vi "AssignAndCount60_Simple.vi"(7 "Area bits in":bool[](array[boolean])=[FALSE, FALSE, FALSE, FALSE, FALSE, FALSE, FALSE, FALSE, FALSE, FALSE, FALSE, FALSE, FALSE, FALSE, FALSE, FALSE, FALSE, FALSE, FALSE, FALSE, FALSE, FALSE, FALSE, FALSE, FALSE, FALSE, FALSE, FALSE, FALSE, FALSE, FALSE, FALSE, FALSE, FALSE, FALSE, FALSE, FALSE, FALSE, FALSE, FALSE, FALSE, FALSE, FALSE, FALSE, FALSE, FALSE, FALSE, FALSE, FALSE, FALSE, FALSE, FALSE, FALSE, FALSE, FALSE, FALSE, FALSE, FALSE, FALSE, FALSE], 9 "PMT bits in":bool[](array[boolean])=[FALSE, FALSE, FALSE, FALSE, FALSE, FALSE, FALSE, FALSE, FALSE, FALSE, FALSE, FALSE, FALSE, FALSE, FALSE, FALSE, FALSE, FALSE, FALSE, FALSE, FALSE, FALSE, FALSE, FALSE, FALSE, FALSE, FALSE, FALSE, FALSE, FALSE, FALSE, FALSE, FALSE, FALSE, FALSE, FALSE, FALSE, FALSE, FALSE, FALSE, FALSE, FALSE, FALSE, FALSE, FALSE, FALSE, FALSE, FALSE, FALSE, FALSE, FALSE, FALSE, FALSE, FALSE, FALSE, FALSE, FALSE, FALSE, FALSE, FALSE], 10 "Photon counter area 2 in":u16, 11 "Photon counter area 1 in":u16) -> (2 "Photon counter area 2 out":u16, 3 "Photon counter area 1 out":u16)   [LabVIEW 2012]
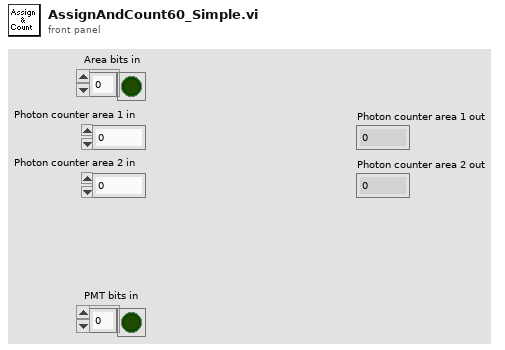
[diagram p1: front panel]
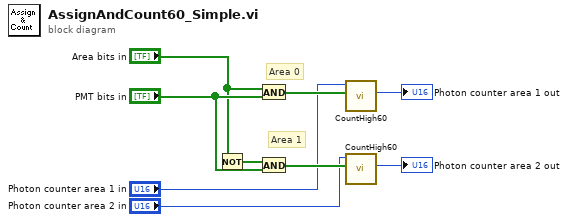
[diagram p0: block diagram]
diagram:
  # "Area 1"
  # "Area 0"
  n1 = Not(x="Area bits in") -> (.not. x?=w9:bool[])
  n2 = And(x="Area bits in", y="PMT bits in") -> (x .and. y?=w7:bool[])
  n3 = And(x=w9, y="PMT bits in") -> (x .and. y?=w6:bool[])
  n4 = call "CountHigh60.vi"("60bit input"=w7, "Previous high count"="Photon counter area 1 in") -> ("New high count"=→"Photon counter area 1 out":u16)  [unwired: 9 in]
  n5 = call "CountHigh60.vi"("60bit input"=w6, "Previous high count"="Photon counter area 2 in") -> ("New high count"=→"Photon counter area 2 out":u16)  [unwired: 9 in]
